vi "Get Calibration Coefficients.vi"(11 "Channel Settings":T1) -> (0 "Zero Value":dbl, 1 "Excitation Voltage":dbl, 2 "Calibration Factor":dbl)   [LabVIEW 2021, in "Acquisition.lvlib"]
doc: "Get the calibration coefficients from 'Channel Settings'."
uses:
  Acquisition.lvlib
  Channel Settings.ctl
  IO Device.ctl
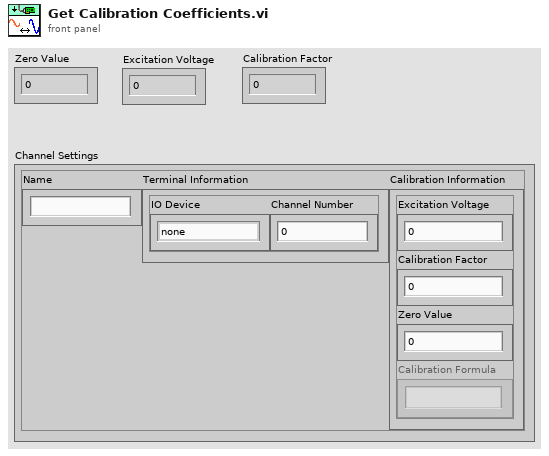
[diagram p1: front panel]
types:
  T1 = typedef "Acquisition.lvlib/Channel Settings.ctl" = cluster{"Name":string, "Terminal Information":cluster{"IO Device":T2, "Channel Number":i32}, "Calibration Information":cluster{"Excitation Voltage":dbl, "Calibration Factor":dbl, "Zero Value":dbl, "Calibration Formula":string}}
  T2 = typedef "Acquisition.lvlib/IO Device.ctl" = enum16{"none", "9219", "9401"}
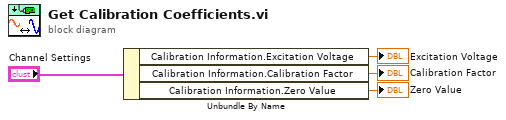
[diagram p0: block diagram]
diagram:
  n1 = Unbundle By Name("Channel Settings") -> ("Calibration Information.Excitation Voltage"=→"Excitation Voltage":dbl, "Calibration Information.Calibration Factor"=→"Calibration Factor":dbl, "Calibration Information.Zero Value"=→"Zero Value":dbl)
